vi "cw_1_4.vi"() -> ()   [LabVIEW 2022 SP3]
panel:
  in  "Farenheit":dbl
  in  "Celcius":dbl
  in  "Enum":enum16{"F -> C", "C -> F"}(ring)
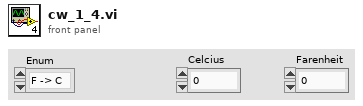
[diagram p1: front panel]
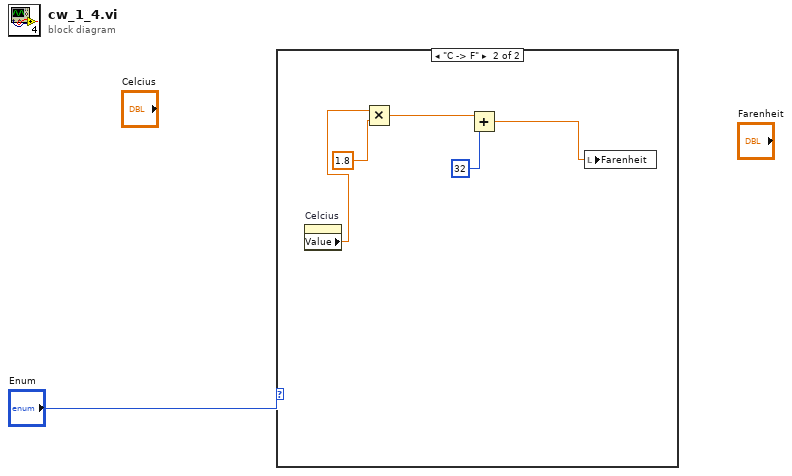
[diagram p0: block diagram]
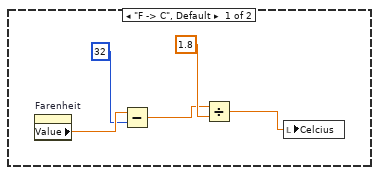
[diagram p2: hidden frame]
diagram:
  n1 = case shown="\"C -> F\"" "Enum" {
    frame "F -> C", Default {
      n2 = property on="Farenheit" class="DigNum (strict)"() -> ("Value"=w6:dbl)  [unwired: 2 in, 2 out]
      n3 = Subtract(x=w6, y=32) -> (x-y=w3:dbl)
      n4 = Divide(x=w3, y=1.8) -> (x/y=w2:dbl)
      n5 = local write "Celcius"(w2) -> ()
    }
    frame "C -> F" {
      n6 = property on="Celcius" class="DigNum (strict)"() -> ("Value"=w8:dbl)  [unwired: 2 in, 2 out]
      n7 = Multiply(x=w8, y=1.8) -> (x*y=w10:dbl)
      n8 = Add(x=w10, y=32) -> (x+y=w7:dbl)
      n9 = local write "Farenheit"(w7) -> ()
    }
  }
